vi "Measures of Spread.vi"(10 "type":i32(ring) items=["standard deviation", "range", "mean absolute deviation", "interquartile range"], 11 "x array":dbl[](array[numeric])) -> (0 "error":i32, 3 "spread value":dbl)   [LabVIEW 2017, in "NI_Gmath.lvlib"]
doc: "Computes the spread of the data values in <B>x array</B>."
uses:
  NI_Gmath.lvlib
  Mean (DBL).vi
  NI_AALBase.lvlib
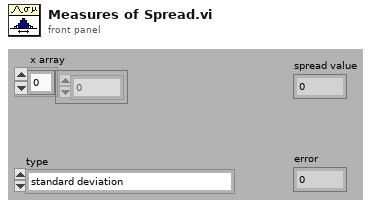
[diagram p1: front panel]
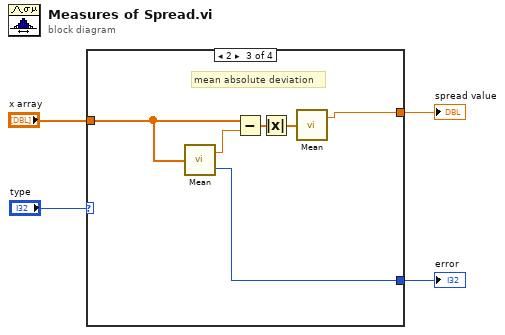
[diagram p0: block diagram]
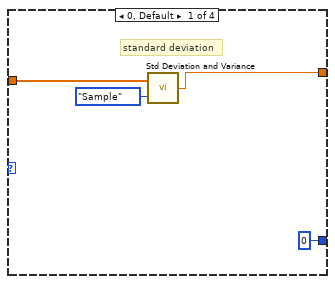
[diagram p2: hidden frame]
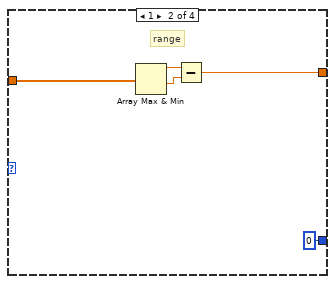
[diagram p3: hidden frame]
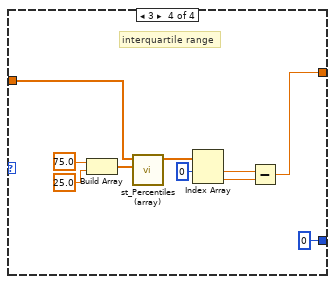
[diagram p4: hidden frame]
diagram:
  n1 = case shown="2" "type" {
    tunnel: "x array" -> [w8 w12 w19 w28]
    tunnel: [w6 w9 w16 w20] -> w2
    tunnel: [0 ("error") 0 ("error") w15 0 ("error")] -> w1
    frame 0, Default {
      # "standard deviation"
      n2 = call "Std Deviation and Variance.vi"("X"=w8, "Weighting (Sample)"=enum16{"Sample", "Population"}."Sample") -> ("standard deviation"=w6:dbl)  [unwired: 2 out]
    }
    frame 1 {
      # "range"
      n3 = Array Max & Min(array=w12) -> (max value=w11:dbl, min value=w10:dbl)  [unwired: 2 out]
      n4 = Subtract(x=w11, y=w10) -> (x-y=w9:dbl)
    }
    frame 2 {
      # "mean absolute deviation"
      n5 = call-poly "Mean.vi"("X"=w19) -> ("mean"=w18:dbl, "error"=w15:i32)
      n6 = Subtract(x=w19, y=w18) -> (x-y=w17:dbl[])
      n7 = Absolute Value(x=w17) -> (abs(x)=w14:dbl[])
      n8 = call-poly "Mean.vi"("X"=w14) -> ("mean"=w16:dbl)  [unwired: 1 out]
    }
    frame 3 {
      # "interquartile range"
      n9 = Build Array(75.0, 25.0) -> (w23:dbl[])
      n10 = call "st_Percentiles (array).vi"("p array"=w23, "x array"=w28) -> ("percentiles"=w27:dbl[])  [unwired: 8 in, 1 out]
      n11 = Index Array(array=w27, index #1=0 ("index")) -> (element #1=w22:dbl, element #2=w21:dbl)  [unwired: 1 in]
      n12 = Subtract(x=w22, y=w21) -> (x-y=w20:dbl)
    }
  }
  "spread value" <- w2
  "error" <- w1
